vi "Loop_SEN.vi"() -> ()   [LabVIEW 2016, in "Controller.lvlib"]
uses:
  Controller.lvlib
  <vilib>/Rock Robotics/WPI/Joystick/WPI_JoystickDeviceEnum.ctl
  Globals/Global_STOP.vi
  Global_Joystick Write_Data.vi
panel:
  out "POVs":i16[](array[numeric])
  out "Buttons":bool[](array[boolean])
  out "Axes":dbl[](array[numeric])
  out "Cycle Time (S)":dbl format="%.3g"
  in  "Target Time(ms)":u32=50
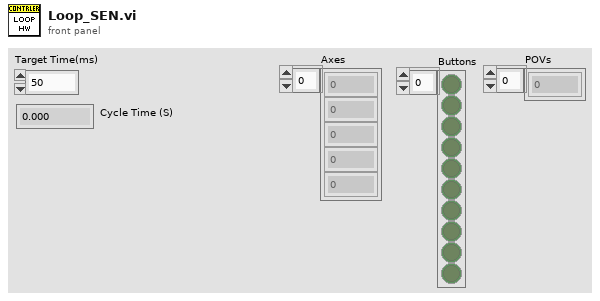
[diagram p1: front panel]
types:
  T1 = typedef "WPI_JoystickDeviceEnum.ctl" = enum16{"USB 0", "USB 1", "USB 2", "USB 3", "USB 4", "USB 5"}
  T2 = typedef "WPI_JoystickDevRef.ctl" = cluster{"Device":T1}
  T3 = cluster{"JoystickDevRef":T2, "Axes":dbl[], "Buttons":bool[], "POVs":i16[], "Target Time(ms)":u32, "Current Time":timestamp, "Previous Time":timestamp, "Cycle Time (S)":dbl}
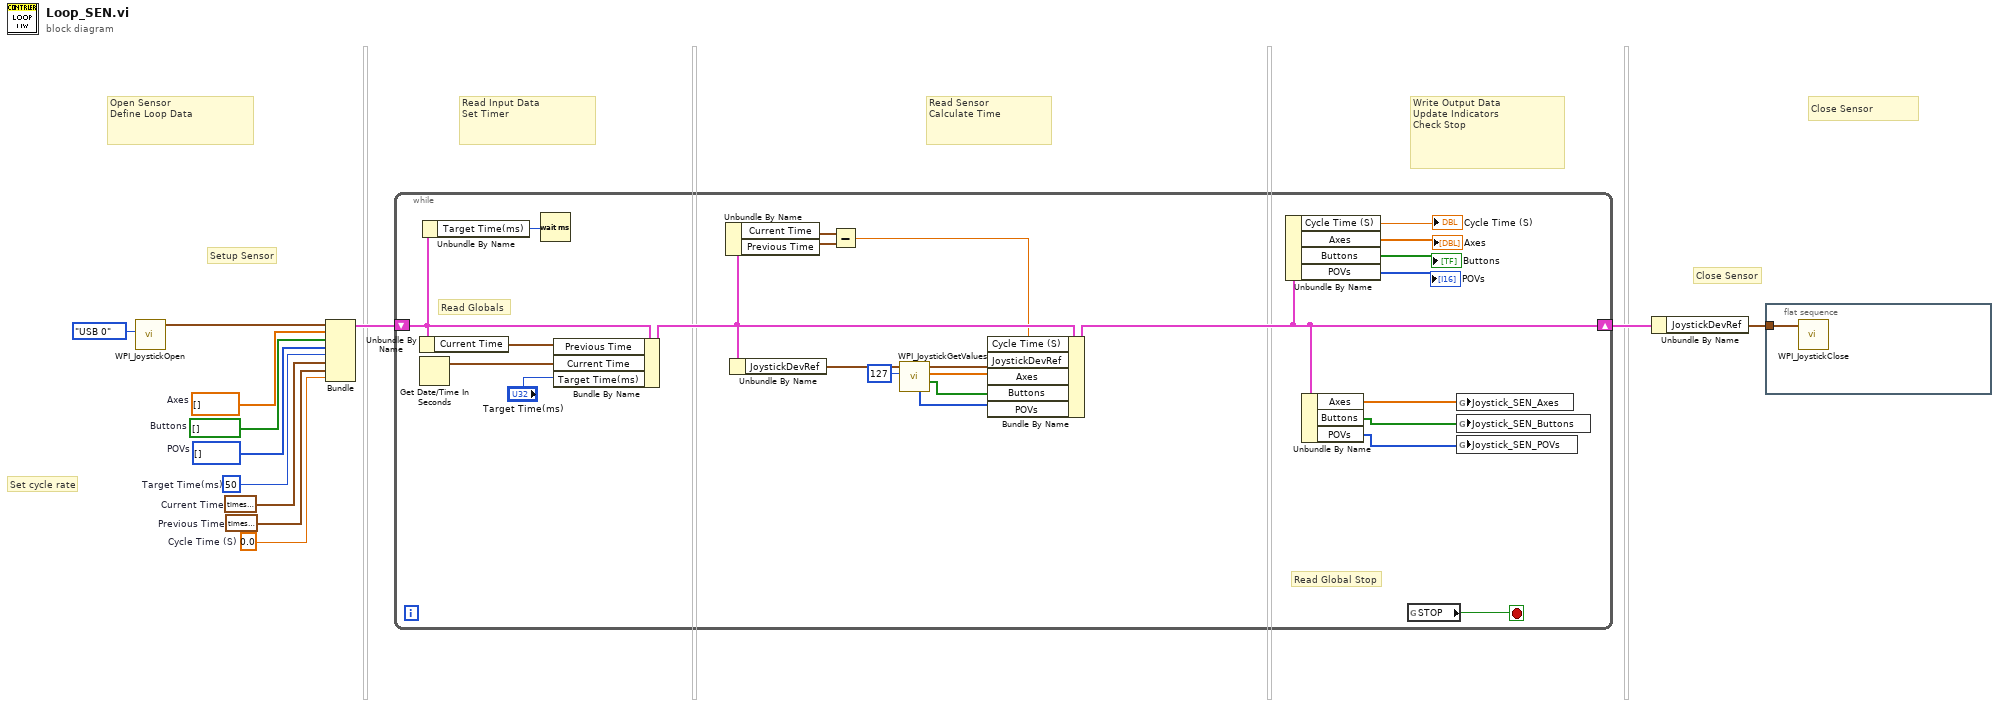
[diagram p0: block diagram]
diagram:
  w2 = i16[] []  # POVs
  w3 = bool[] []  # Buttons
  w4 = dbl[] []  # Axes
  w5 = 0.0  # Cycle Time (S)
  w12 = timestamp(0 s since 1904-01-01)  # Previous Time
  w11 = timestamp(0 s since 1904-01-01)  # Current Time
  w10 = u32 50  # Target Time(ms)
  # "Close Sensor"
  # "Write Output Data\nUpdate Indicators\nCheck Stop"
  # "Read Sensor\nCalculate Time"
  # "Read Input Data\nSet Timer"
  # "Open Sensor\nDefine Loop Data"
  # "Set cycle rate"
  # "Close Sensor"
  # "Setup Sensor"
  n1 = call <vilib>:"WPI_JoystickOpen.vi"("JoystickDevice"=WPI_JoystickDeviceEnum."USB 0") -> ("JoystickDevRef"=w7:T2)  [unwired: 10 in]
  n2 = Bundle("JoystickDevRef"=w7, "Axes"=w4, "Buttons"=w3, "POVs"=w2, "Target Time(ms)"=w10, "Current Time"=w11, "Previous Time"=w12, "Cycle Time (S)"=w5) -> (w8:T3)  [unwired: 1 in]
  n3 = while {
    shift-right: [w24] -> w6
    shift-left: w8 -> [w26]
    stop <- w36 stop-if-true
    # "Read Globals"
    # "Read Global Stop"
    n4 = Unbundle By Name(w26) -> ("Current Time"=w31:timestamp)
    n5 = Get Date/Time In Seconds() -> (seconds since 1Jan1904=w32:timestamp)
    n6 = Unbundle By Name(w26) -> ("Target Time(ms)"=w25:u32)
    n7 = Wait (ms)(milliseconds to wait=w25) -> ()  [unwired: 1 out]
    n8 = Bundle By Name(cluster=w26, "Previous Time"=w31, "Current Time"=w32, "Target Time(ms)"="Target Time(ms)") -> (w27:T3)
    n9 = Unbundle By Name(w27) -> ("Current Time"=w30:timestamp, "Previous Time"=w29:timestamp)
    n10 = Unbundle By Name(w27) -> ("JoystickDevRef"=w35:T2)
    n11 = Subtract(x=w30, y=w29) -> (x-y=w22:dbl)
    n12 = call <vilib>:"WPI_JoystickGetValues.vi"("Scaler"=i8 127, "JoystickDevRef"=w35) -> ("Buttons"=w20:bool[], "Axes"=w21:dbl[], "JoystickDevRef"=w34:T2, "POVs"=w19:i16[])  [unwired: 5 in, 1 out]
    n13 = Bundle By Name(cluster=w27, "Cycle Time (S)"=w22, "JoystickDevRef"=w34, "Axes"=w21, "Buttons"=w20, "POVs"=w19) -> (w24:T3)
    n14 = Unbundle By Name(w24) -> ("Cycle Time (S)"=→"Cycle Time (S)":dbl, "Axes"=→"Axes":dbl[], "Buttons"=→"Buttons":bool[], "POVs"=→"POVs":i16[])
    n15 = Unbundle By Name(w24) -> ("Axes"=w33:dbl[], "Buttons"=w15:bool[], "POVs"=w14:i16[])
    n16 = global read "Global_STOP.vi" "STOP"() -> (w36:bool)
    n17 = global write "Global_Joystick Write_Data.vi" "Joystick_SEN_Axes"(w33) -> ()
    n18 = global write "Global_Joystick Write_Data.vi" "Joystick_SEN_Buttons"(w15) -> ()
    n19 = global write "Global_Joystick Write_Data.vi" "Joystick_SEN_POVs"(w14) -> ()
  }
  n20 = Unbundle By Name(w6) -> ("JoystickDevRef"=w9:T2)
  n21 = flat-sequence {
    tunnel: w9 -> [w37]
    frame #0 {
      n22 = call <vilib>:"WPI_JoystickClose.vi"("JoystickDevRef"=w37) -> ()  [unwired: 11 in]
    }
  }
